vi "Close-connection.vi"(8 "error in (no error)":errorcluster, 11 "SM1000-control in":T1) -> (0 "error out":errorcluster, 1 "Closed?":bool, 3 "SM1000-control out":T1)   [LabVIEW 2013, in "HardwareCharacterization.lvlib" / "HC-SM1000.lvclass"]
uses:
  HC-SM1000.lvclass
  Object-reference.ctl
  HC-SM1000.lvclass/HC-SM1000.ctl
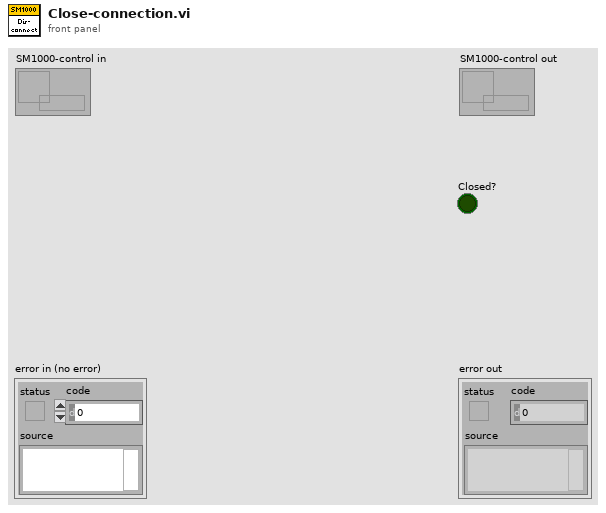
[diagram p1: front panel]
types:
  T1 = typedef "HardwareCharacterization.lvlib/HC-SM1000.lvclass/Object-reference.ctl" = refnum<data-value>
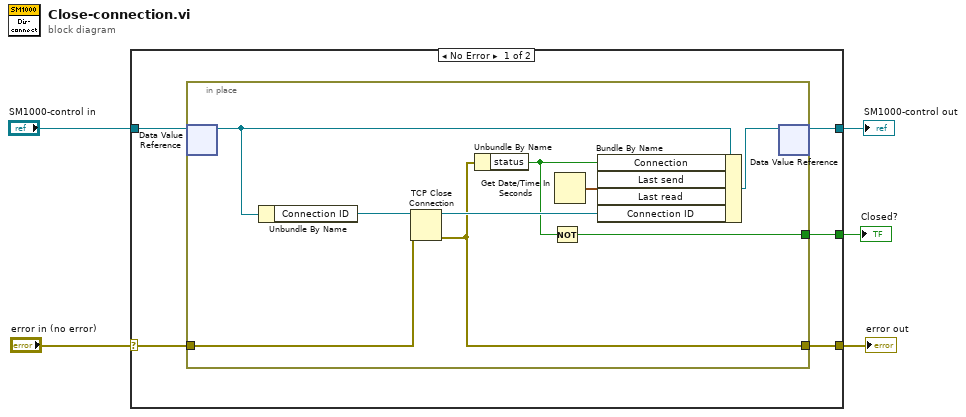
[diagram p0: block diagram]
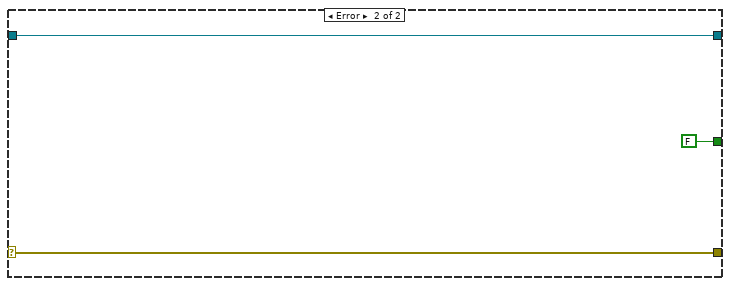
[diagram p2: hidden frame]
diagram:
  n1 = case shown="No Error" "error in (no error)" {
    selector: "error in (no error)" -> [w8 w22]
    tunnel: [w7 w22] -> w4
    tunnel: [w9 w21] -> w2
    tunnel: "SM1000-control in" -> [w10 w21]
    tunnel: [w6 FALSE] -> w1
    frame No Error {
      n2 = in-place {
        in-place-border: w8 -> [w19]
        in-place-border: [w13] -> w7
        in-place-border: [w11] -> w6
        n3 = in-place-dvr #1(w10) -> (w18:refnum<class "HC-SM1000.lvclass">)  [unwired: 1 out]
        n4 = Unbundle By Name(w18) -> ("Connection ID"=w14:refnum<k5>)
        n5 = TCP Close Connection(connection ID=w14, error in (no error)=w19) -> (connection ID out=w17:refnum<k5>, error out=w13:errorcluster)  [unwired: 1 in]
        n6 = Unbundle By Name(w13) -> ("status"=w12:bool)
        n7 = Not(x=w12) -> (.not. x?=w11:bool)
        n8 = Get Date/Time In Seconds() -> (seconds since 1Jan1904=w16:timestamp)
        n9 = Bundle By Name(cluster=w18, "Connection"=w12, "Last send"=w16, "Last read"=w16, "Connection ID"=w17) -> (w15:refnum<class "HC-SM1000.lvclass">)
        n10 = in-place-dvr #1(w15) -> (w9:T1)  [unwired: 1 out]
      }
    }
    frame Error {
    }
  }
  "error out" <- w4
  "SM1000-control out" <- w2
  "Closed?" <- w1
